vi "LIA7230_Manage_Monitor.vi"(3 "Lock -In # (in)":i32, 4 "System Monitor Variables (in)":T2, 5 "Command- (in)":T1={"Lockin 1"=[], "X1-Display"=0.0, "X1 Percent"=0.0, "Y1-Display"=0.0, "X1 Percent 2"=0.0, "Unit X1"="nV", "Unit X2"="nV", "X1 Overload"=FALSE, "Y1 Overload"=FALSE, "Sensitivity Setpoint"=26, "X1"=0.0, "Y1"=0.0, "Channel 3"=0.0, "Channel 4"=0.0, "Channel 4 Percent"=0.0, "Channel 3 Percent "=0.0, "Unit Channel 3"="nV", "Unit Channel 4"="nV", "Overload channel 3"=FALSE, "Overload channel 4"=FALSE, "Offsets (ON)"=FALSE, "Sensitivity Setpoint 2"=26} {"Sensitivity Setpoint 2" items=["2 nV", "5 nV", "10 nV", "20 nV", "50 nV", "100 nV", "200 nV", "500 nV", "1 µV", "2 µV", "5 µV", "10 µV", "20 µV", "50 µV", "100 µV", "200 µV", "500 µV", "1 mV", "2 mV", "5 mV", "10 mV", "20 mV", "50 mV", "100 mV", "200 mV", "500 mV", "1 V", ""]; "Channel 3 Percent" scale=0.0..1.0; "Channel 4 Percent" scale=0.0..1.0; "Sensitivity Setpoint" items=["2 nV", "5 nV", "10 nV", "20 nV", "50 nV", "100 nV", "200 nV", "500 nV", "1 µV", "2 µV", "5 µV", "10 µV", "20 µV", "50 µV", "100 µV", "200 µV", "500 µV", "1 mV", "2 mV", "5 mV", "10 mV", "20 mV", "50 mV", "100 mV", "200 mV", "500 mV", "1 V", ""]; "X1 Percent 2" scale=0.0..1.0; "X1 Percent" scale=0.0..1.0; "X1-Display" format="%#4_5f"}, 6 "Global Status (in)":T1={"Lockin 1"=[], "X1-Display"=0.0, "X1 Percent"=0.0, "Y1-Display"=0.0, "X1 Percent 2"=0.0, "Unit X1"="nV", "Unit X2"="nV", "X1 Overload"=FALSE, "Y1 Overload"=FALSE, "Sensitivity Setpoint"=26, "X1"=0.0, "Y1"=0.0, "Channel 3"=0.0, "Channel 4"=0.0, "Channel 4 Percent"=0.0, "Channel 3 Percent "=0.0, "Unit Channel 3"="nV", "Unit Channel 4"="nV", "Overload channel 3"=FALSE, "Overload channel 4"=FALSE, "Offsets (ON)"=FALSE, "Sensitivity Setpoint 2"=26} {"Sensitivity Setpoint 2" items=["2 nV", "5 nV", "10 nV", "20 nV", "50 nV", "100 nV", "200 nV", "500 nV", "1 µV", "2 µV", "5 µV", "10 µV", "20 µV", "50 µV", "100 µV", "200 µV", "500 µV", "1 mV", "2 mV", "5 mV", "10 mV", "20 mV", "50 mV", "100 mV", "200 mV", "500 mV", "1 V", ""]; "Channel 3 Percent" scale=0.0..1.0; "Channel 4 Percent" scale=0.0..1.0; "Sensitivity Setpoint" items=["2 nV", "5 nV", "10 nV", "20 nV", "50 nV", "100 nV", "200 nV", "500 nV", "1 µV", "2 µV", "5 µV", "10 µV", "20 µV", "50 µV", "100 µV", "200 µV", "500 µV", "1 mV", "2 mV", "5 mV", "10 mV", "20 mV", "50 mV", "100 mV", "200 mV", "500 mV", "1 V", ""]; "X1 Percent 2" scale=0.0..1.0; "X1 Percent" scale=0.0..1.0; "X1-Display" format="%#4_5f"}, 7 "queue (in)":refnum<queue>) -> (0 "Monitor (out)":T1={"Lockin 1"=[], "X1-Display"=0.0, "X1 Percent"=0.0, "Y1-Display"=0.0, "X1 Percent 2"=0.0, "Unit X1"="nV", "Unit X2"="nV", "X1 Overload"=FALSE, "Y1 Overload"=FALSE, "Sensitivity Setpoint"=26, "X1"=0.0, "Y1"=0.0, "Channel 3"=0.0, "Channel 4"=0.0, "Channel 4 Percent"=0.0, "Channel 3 Percent "=0.0, "Unit Channel 3"="nV", "Unit Channel 4"="nV", "Overload channel 3"=FALSE, "Overload channel 4"=FALSE, "Offsets (ON)"=FALSE, "Sensitivity Setpoint 2"=26} {"Sensitivity Setpoint 2" items=["2 nV", "5 nV", "10 nV", "20 nV", "50 nV", "100 nV", "200 nV", "500 nV", "1 µV", "2 µV", "5 µV", "10 µV", "20 µV", "50 µV", "100 µV", "200 µV", "500 µV", "1 mV", "2 mV", "5 mV", "10 mV", "20 mV", "50 mV", "100 mV", "200 mV", "500 mV", "1 V", ""]; "Channel 3 Percent" scale=0.0..1.0; "Channel 4 Percent" scale=0.0..1.0; "Sensitivity Setpoint" items=["2 nV", "5 nV", "10 nV", "20 nV", "50 nV", "100 nV", "200 nV", "500 nV", "1 µV", "2 µV", "5 µV", "10 µV", "20 µV", "50 µV", "100 µV", "200 µV", "500 µV", "1 mV", "2 mV", "5 mV", "10 mV", "20 mV", "50 mV", "100 mV", "200 mV", "500 mV", "1 V", ""]; "X1 Percent 2" scale=0.0..1.0; "X1 Percent" scale=0.0..1.0; "X1-Display" format="%#4_5f"}, 1 "System Monitor Variables (out)":T2)   [LabVIEW 2019]
uses:
  Global/Global Variables/System Monitor Cluster.ctl
  LIA7230/LIA7230-cluster.ctl
  Instrument_Setup.vi
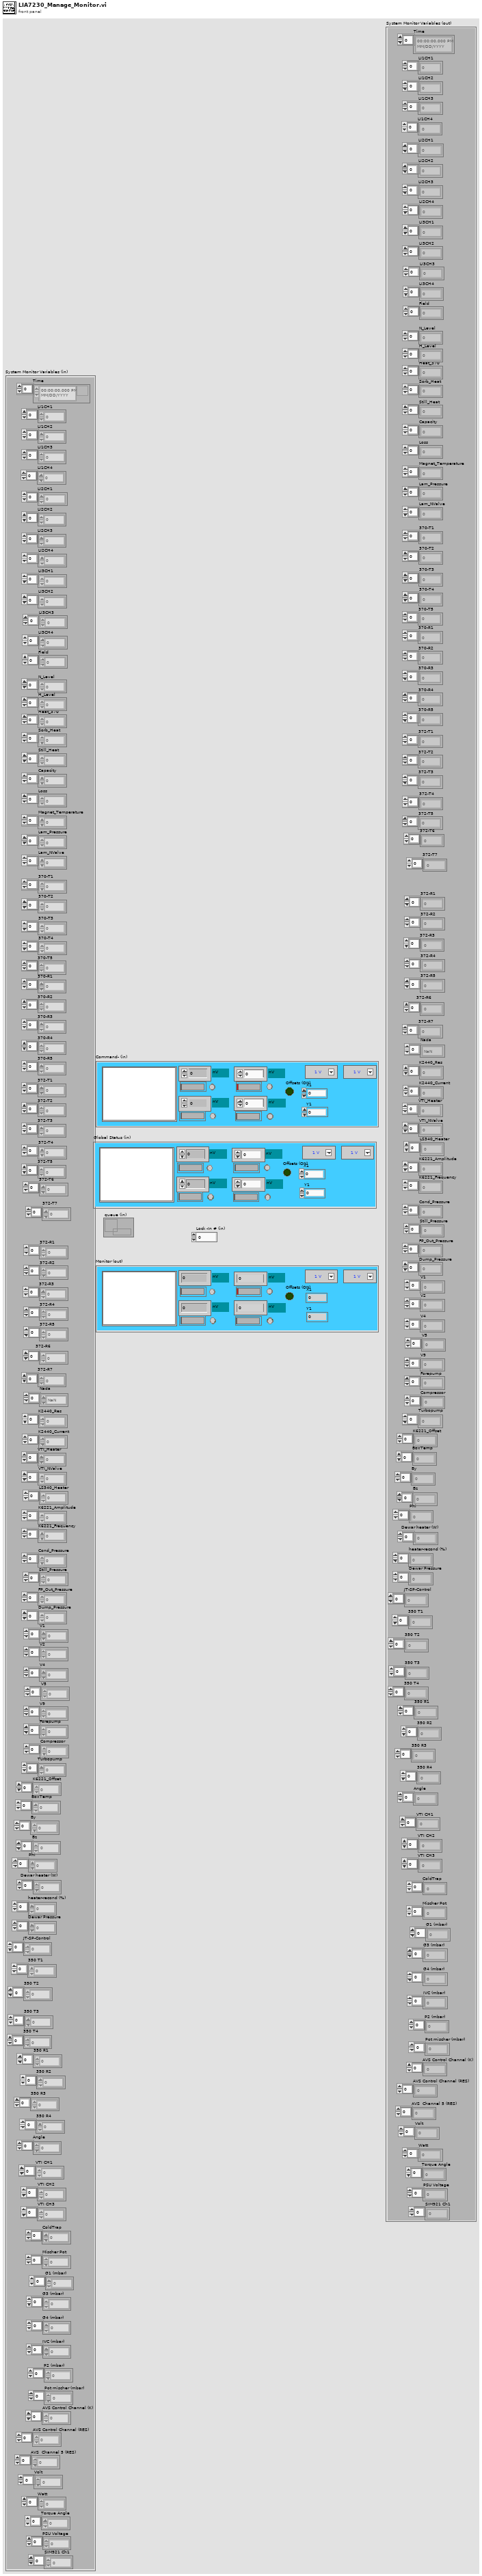
[diagram p1: front panel]
types:
  T1 = typedef "LIA7230-cluster.ctl" = cluster{"Lockin 1":dbl[][], "X1-Display":dbl, "X1 Percent":dbl, "Y1-Display":dbl, "X1 Percent 2":dbl, "Unit X1":string, "Unit X2":string, "X1 Overload":bool, "Y1 Overload":bool, "Sensitivity Setpoint":i16, "X1":dbl, "Y1":dbl, "Channel 3":dbl, "Channel 4":dbl, "Channel 4 Percent":dbl, "Channel 3 Percent ":dbl, "Unit Channel 3":string, "Unit Channel 4":string, "Overload channel 3":bool, "Overload channel 4":bool, "Offsets (ON)":bool, "Sensitivity Setpoint 2":i16}
  T2 = typedef "System Monitor Cluster.ctl" = cluster{"Time":timestamp[], "LI1CH1":dbl[], "LI1CH2":dbl[], "LI2CH1":dbl[], "LI2CH2":dbl[], "LI3CH1":dbl[], "LI3CH2":dbl[], "Field":dbl[], "N_Level":dbl[], "H_Level":dbl[], "Heat_370":dbl[], "Sorb_Heat":dbl[], "Still_Heat":dbl[], "Capacity":dbl[], "Loss":dbl[], "Magnet_Temperature":dbl[], "Lam_Pressure":dbl[], "Lam_NValve":dbl[], "370-T1":dbl[], "370-T2":dbl[], "370-T3":dbl[], "370-T4":dbl[], "370-T5":dbl[], "370-R1":dbl[], "370-R2":dbl[], "370-R3":dbl[], "370-R4":dbl[], "370-R5":dbl[], "372-T1":dbl[], "372-T2":dbl[], "372-T3":dbl[], "372-T4":dbl[], "372-T5":dbl[], "372-T6":dbl[], "372-R1":dbl[], "372-R2":dbl[], "372-R3":dbl[], "372-R4":dbl[], "372-R5":dbl[], "372-R6":dbl[], "Nada":dbl[], "K2440_Res":dbl[], "K2440_Current":dbl[], "VTI_Heater":dbl[], "VTI_NValve":dbl[], "LS340_Heater":dbl[], "K6221_Amplitude":dbl[], "K6221_Frequency":dbl[], "Cond_Pressure":dbl[], "Still_Pressure":dbl[], "FP_Out_Pressure":dbl[], "Dump_Pressure":dbl[], "V1":dbl[], "V2":dbl[], "V4":dbl[], "V5":dbl[], "V9":dbl[], "Forepump":dbl[], "Compressor":dbl[], "K6221_Offset":dbl[], "BoxTemp":dbl[], "By":dbl[], "Bz":dbl[], "Phi":dbl[], "heater-recond (%)":dbl[], "Dewar Pressure ":dbl[], "JT-SP-Control":dbl[], "350 T1":dbl[], "350 T2":dbl[], "350 T3":dbl[], "350 T4":dbl[], "350 R1":dbl[], "350 R2":dbl[], "350 R3":dbl[], "350 R4":dbl[], "Angle":dbl[], "VTI CH1":dbl[], "VTI CH2":dbl[], "VTI CH3":dbl[], "ColdTrap":dbl[], "Mischer Pot":dbl[], "G1 (mbar)":dbl[], "G3 (mbar) ":dbl[], "G4 (mbar)":dbl[], "IVC (mbar)":dbl[], "P2 (mbar) ":dbl[], "Pot mischer (mbar)":dbl[], "AVS Control Channel (K)":dbl[], "AVS Control Channel (RES)":dbl[], "AVS  Channel 5 (RES) ":dbl[], "LI3CH3":dbl[], "LI3CH4":dbl[], "LI1CH3":dbl[], "LI1CH4":dbl[], "LI2CH3":dbl[], "LI2CH4":dbl[], "Volt":dbl[], "Watt":dbl[], "Torque Angle":dbl[], "Dewar heater (W)":dbl[], "PSU Voltage":dbl[], "Turbopump":dbl[], "372-R7":dbl[], "372-T7":dbl[], "SIM921 Ch1":dbl[]}
  T3 = cluster{"Interface":u16, "Port":u16, "Serial Number":string, "IP Address":string, "Line Frequency\nRejection Filter":u8, "Input Mode":u16, "Input Conn. Shells":bool, "Line Frequency":bool, "Auto AC Gain":bool, "AC Gain":u16, "Input Device":bool, "Range":u8, " Auto Sensitivity ":bool, "Auto Measure":bool, "Range 2":u8, " Auto Sensitivity  2":bool, "Slope":u8, "Synchronous TC":bool, "Time Constant":u16, "Slope 2":u8, "Time Constant 2":u16, "Oscillator Amp (V rms)":dbl, "Oscillator Freq (Hz)":dbl, "Reference I/P":u8, "Ref Harm 1":u16, "Ref Harm2":u16, "Virtual Ref.\nMode":bool, "Dual Harmonic/Reference Mode":bool, "Reference Mode":bool, "TRIG OUT\n= Ref Mon":bool, " Auto Phase ":bool, "Reference Phase 1":dbl, "+90 degrees 1":bool, " Auto Phase 2 ":bool, "Reference 2 Phase":dbl, "+90 degrees2":bool, "Auxiliary I/O":bool, "Configuration":bool, "Curve Buffer":bool, "Offsets":bool, "X Channel Offset (%)":sgl, "X Channel Offset":bool, "Y Channel Offset (%)":dbl, "Y Channel Offset":bool, " Auto Offset":bool, "X Channel Offset (%) 2":sgl, "X Channel Offset 2":bool, "Y Channel Offset (%) 2":dbl, "Y Channel Offset 2":bool, " Auto Offset 2":bool, "Display Type channel 1":u16, "Display Type channel 2":u16, "Display Type channel 3":u16, "Display Type channel 4":u16, "Osc Sweeps":bool, "Define Equation1":bool, "Coupling":bool}
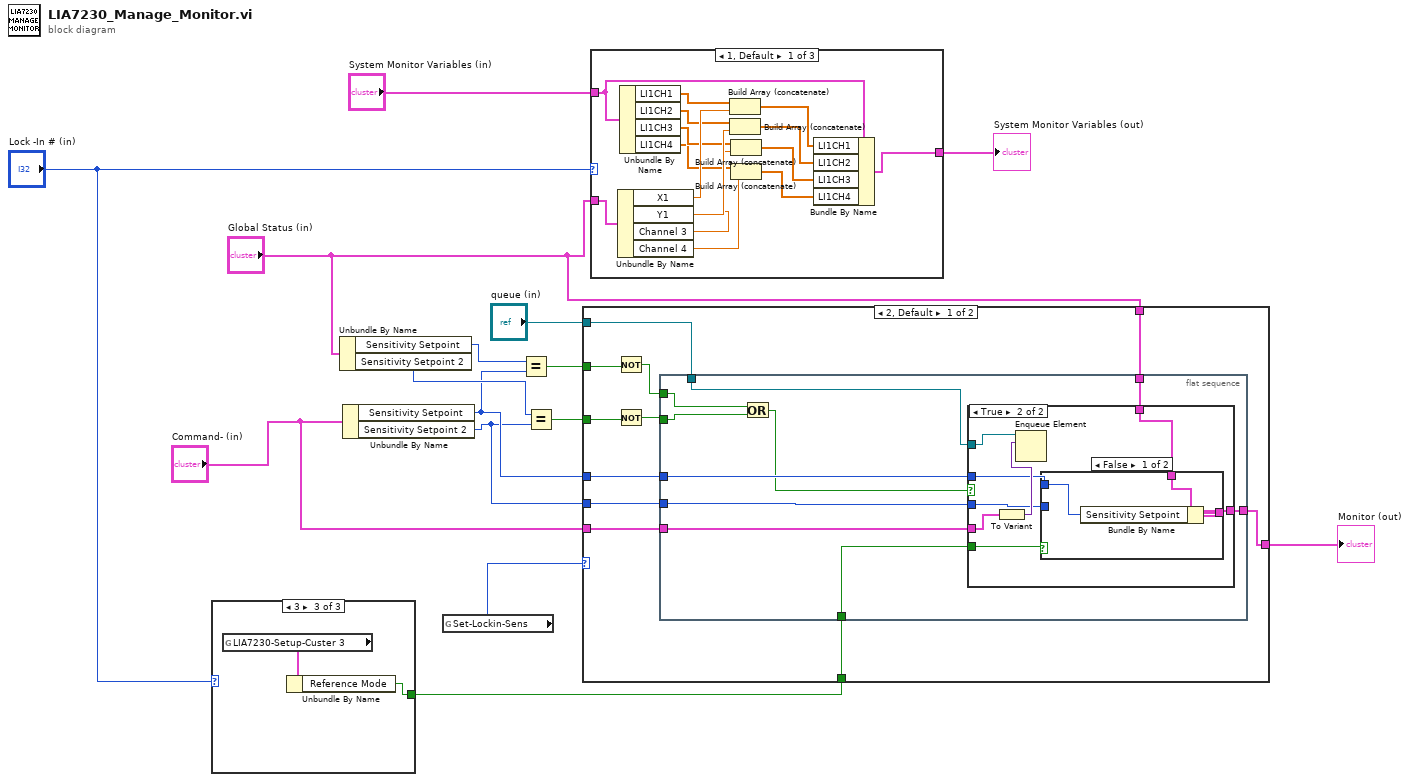
[diagram p0: block diagram]
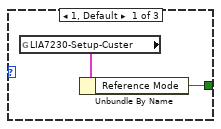
[diagram p2: hidden frame]
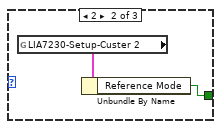
[diagram p3: hidden frame]
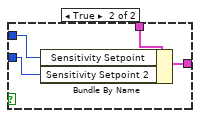
[diagram p5: hidden frame]
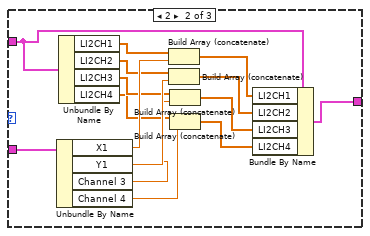
[diagram p7: hidden frame]
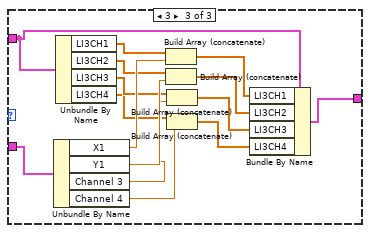
[diagram p8: hidden frame]
diagram:
  n1 = case shown="3" "Lock -In # (in)" {
    tunnel: [w16 w18 w20] -> w1
    frame 1, Default {
      n2 = global read "Instrument_Setup.vi" "LIA7230-Setup-Custer"() -> (w17:T3)
      n3 = Unbundle By Name(w17) -> ("Reference Mode"=w16:bool)
    }
    frame 2 {
      n4 = global read "Instrument_Setup.vi" "LIA7230-Setup-Custer 2"() -> (w19:T3)
      n5 = Unbundle By Name(w19) -> ("Reference Mode"=w18:bool)
    }
    frame 3 {
      n6 = global read "Instrument_Setup.vi" "LIA7230-Setup-Custer 3"() -> (w21:T3)
      n7 = Unbundle By Name(w21) -> ("Reference Mode"=w20:bool)
    }
  }
  n8 = Unbundle By Name("Global Status (in)") -> ("Sensitivity Setpoint"=w9:i16, "Sensitivity Setpoint 2"=w8:i16)
  n9 = Unbundle By Name("Command- (in)") -> ("Sensitivity Setpoint"=w4:i16, "Sensitivity Setpoint 2"=w3:i16)
  n10 = global read "Instrument_Setup.vi" "Set-Lockin-Sens"() -> (w13:u16)
  n11 = Equal?(x=w9, y=w4) -> (x = y?=w7:bool)
  n12 = Equal?(x=w8, y=w3) -> (x = y?=w6:bool)
  n13 = case shown="2, Default" w13 {
    tunnel: "Global Status (in)" -> [w28 w59]
    tunnel: [w27 w59] -> w12
    tunnel: "Command- (in)" -> [w31 _]
    tunnel: w7 -> [w26 _]
    tunnel: w6 -> [w25 _]
    tunnel: "queue (in)" -> [w32 _]
    tunnel: w4 -> [w30 _]
    tunnel: w3 -> [w29 _]
    tunnel: w1 -> [w22 _]
    frame 2, Default {
      n14 = Not(x=w26) -> (.not. x?=w24:bool)
      n15 = Not(x=w25) -> (.not. x?=w23:bool)
      n16 = flat-sequence {
        tunnel: w32 -> [w40]
        tunnel: w24 -> [w42]
        tunnel: w23 -> [w41]
        tunnel: w31 -> [w39]
        tunnel: w30 -> [w36]
        tunnel: w29 -> [w35]
        tunnel: w28 -> [w38]
        tunnel: [w37] -> w27
        tunnel: w22 -> [w33]
        frame #0 {
          n17 = Or(x=w42, y=w41) -> (x .or. y?=w34:bool)
          n18 = case shown="True" w34 {
            tunnel: w40 -> [_ w51]
            tunnel: w39 -> [_ w50]
            tunnel: w38 -> [w43 w48]
            tunnel: [w43 w47] -> w37
            tunnel: w36 -> [_ w46]
            tunnel: w35 -> [_ w45]
            tunnel: w33 -> [_ w44]
            frame False {
            }
            frame True {
              n19 = To Variant(anything=w50) -> (Variant=w49:variant)
              n20 = Enqueue Element(queue=w51, element=w49) -> ()  [unwired: 2 in, 3 out]
              n21 = case shown="False" w44 {
                tunnel: w48 -> [w54 w58]
                tunnel: [w53 w57] -> w47
                tunnel: w46 -> [w52 w56]
                tunnel: w45 -> [_ w55]
                frame False {
                  n22 = Bundle By Name(cluster=w54, "Sensitivity Setpoint"=w52) -> (w53:T1)
                }
                frame True {
                  n23 = Bundle By Name(cluster=w58, "Sensitivity Setpoint"=w56, "Sensitivity Setpoint 2"=w55) -> (w57:T1)
                }
              }
            }
          }
        }
      }
    }
    frame 0, 1 {
    }
  }
  "Monitor (out)" <- w12
  n24 = case shown="1, Default" "Lock -In # (in)" {
    tunnel: "System Monitor Variables (in)" -> [w62 w80 w91]
    tunnel: "Global Status (in)" -> [w61 w89 w92]
    tunnel: [w60 w79 w90] -> w14
    frame 1, Default {
      n25 = Unbundle By Name(w61) -> ("X1"=w73:dbl, "Y1"=w71:dbl, "Channel 3"=w69:dbl, "Channel 4"=w67:dbl)
      n26 = Unbundle By Name(w62) -> ("LI1CH1"=w74:dbl[], "LI1CH2"=w72:dbl[], "LI1CH3"=w70:dbl[], "LI1CH4"=w68:dbl[])
      n27 = Build Array (concatenate)(w74, w73) -> (w66:dbl[])
      n28 = Build Array (concatenate)(w72, w71) -> (w65:dbl[])
      n29 = Build Array (concatenate)(w70, w69) -> (w64:dbl[])
      n30 = Build Array (concatenate)(w68, w67) -> (w63:dbl[])
      n31 = Bundle By Name(cluster=w62, "LI1CH1"=w66, "LI1CH2"=w65, "LI1CH3"=w64, "LI1CH4"=w63) -> (w60:T2)
    }
    frame 2 {
      n32 = Unbundle By Name(w89) -> ("X1"=w87:dbl, "Y1"=w85:dbl, "Channel 3"=w83:dbl, "Channel 4"=w81:dbl)
      n33 = Unbundle By Name(w80) -> ("LI2CH1"=w88:dbl[], "LI2CH2"=w86:dbl[], "LI2CH3"=w84:dbl[], "LI2CH4"=w82:dbl[])
      n34 = Build Array (concatenate)(w88, w87) -> (w78:dbl[])
      n35 = Build Array (concatenate)(w86, w85) -> (w77:dbl[])
      n36 = Build Array (concatenate)(w84, w83) -> (w76:dbl[])
      n37 = Build Array (concatenate)(w82, w81) -> (w75:dbl[])
      n38 = Bundle By Name(cluster=w80, "LI2CH1"=w78, "LI2CH2"=w77, "LI2CH3"=w76, "LI2CH4"=w75) -> (w79:T2)
    }
    frame 3 {
      n39 = Unbundle By Name(w92) -> ("X1"=w103:dbl, "Y1"=w101:dbl, "Channel 3"=w99:dbl, "Channel 4"=w97:dbl)
      n40 = Unbundle By Name(w91) -> ("LI3CH1"=w104:dbl[], "LI3CH2"=w102:dbl[], "LI3CH3"=w100:dbl[], "LI3CH4"=w98:dbl[])
      n41 = Build Array (concatenate)(w104, w103) -> (w96:dbl[])
      n42 = Build Array (concatenate)(w102, w101) -> (w95:dbl[])
      n43 = Build Array (concatenate)(w100, w99) -> (w94:dbl[])
      n44 = Build Array (concatenate)(w98, w97) -> (w93:dbl[])
      n45 = Bundle By Name(cluster=w91, "LI3CH1"=w96, "LI3CH2"=w95, "LI3CH3"=w94, "LI3CH4"=w93) -> (w90:T2)
    }
  }
  "System Monitor Variables (out)" <- w14
